vi "QTI Sensor.vi"(8 "error in (no error)":errorcluster, 9 "level":dbl, 11 "IIC in":refnum<class "IIC.lvclass">) -> (0 "error out":errorcluster, 1 "QTI Binary":bool[](array[boolean]), 2 "QTI":dbl[](array[numeric]), 3 "IIC out":refnum<class "IIC.lvclass">)   [LabVIEW 2020]
uses:
  <vilib>/High Genius/HG_WSI_Tookit/Dependencies/Library/IIC/IIC.lvclass
  C:/Program Files (x86)/National Instruments/LabVIEW 2020/vi.lib/High Genius/HG_WSI_Tookit/Dependencies/Library/HG_LIB/HG_LIB.lvclass
  <vilib>/High Genius/HG_WSI_Tookit/Dependencies/Library/HG_LIB/HG_LIB.lvclass
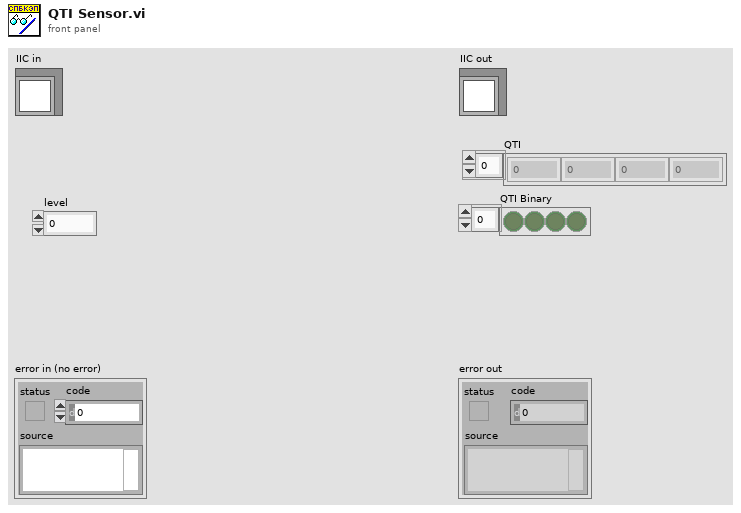
[diagram p1: front panel]
types:
  T1 = cluster{"data":cluster{"ai22":sgl, "ai23":sgl, "ai24":sgl, "ai25":sgl, "pulse12":i32, "pulse13":i32, "pwm14":i32, "pwm15":i32, "pwm16":i32, "do17":bool, "do18":bool, "do19":bool, "do20":bool, "do21":bool, "di11":bool, "di9":bool, "motor0":u8, "motor1":u8, "motor2":u8, "motor3":u8, "dir00":u8, "dir01":u8, "dir02":u8, "dir03":u8, "dir10":u8, "dir11":u8, "dir12":u8, "dir13":u8, "limit0":bool, "limit1":bool, "limit2":bool, "limit3":bool, "limit4":bool, "limit5":bool, "limit6":bool, "limit7":bool, "lsb0H":u8, "lsb1H":u8, "lsb2H":u8, "lsb3H":u8, "lsb0L":u8, "lsb1L":u8, "lsb2L":u8, "lsb3L":u8, "enc0_counters":u32, "enc1_counters":u32, "enc2_counters":u32, "enc3_counters":u32, "counter10":u32, "counter8":u32, "reset_enc0":bool, "reset_enc1":bool, "reset_enc2":bool, "reset_enc3":bool, "pitch":sgl, "roll":sgl, "yaw":sgl, "zero_yaw":bool}}
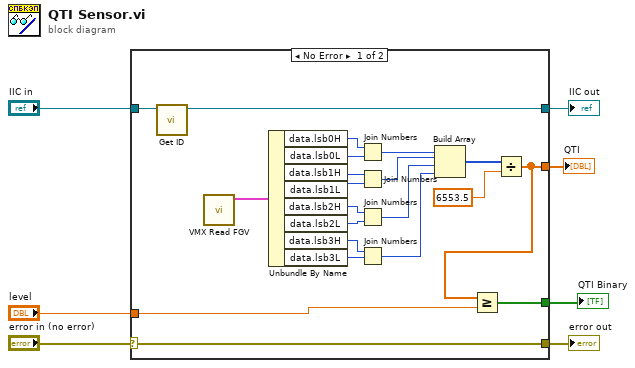
[diagram p0: block diagram]
diagram:
  n1 = case shown="No Error" "error in (no error)" {
    selector: "error in (no error)" -> [w13 w30]
    tunnel: [w13 w30] -> w3
    tunnel: [w28 w29] -> w5
    tunnel: "IIC in" -> [w27 w29]
    tunnel: [w9 _] -> w4
    tunnel: "level" -> [w10 _]
    tunnel: [w8 _] -> w1
    frame No Error {
      n2 = call <vilib>:"Get ID.vi"("HG_LIB in"=w27) -> ("HG_LIB out"=w28:refnum<class "IIC.lvclass">)  [unwired: 9 in, 1 out]
      n3 = call <vilib>:"VMX Read FGV.vi"() -> ("Read Data"=w20:T1)  [unwired: 10 in, 1 out]
      n4 = Unbundle By Name(w20) -> ("data.lsb0H"=w19:u8, "data.lsb0L"=w18:u8, "data.lsb1H"=w17:u8, "data.lsb1L"=w16:u8, "data.lsb2H"=w15:u8, "data.lsb2L"=w14:u8, "data.lsb3H"=w12:u8, "data.lsb3L"=w11:u8)
      n5 = Join Numbers(hi=w19, lo=w18) -> ((hi.lo)=w26:u16)
      n6 = Join Numbers(hi=w17, lo=w16) -> ((hi.lo)=w25:u16)
      n7 = Join Numbers(hi=w15, lo=w14) -> ((hi.lo)=w24:u16)
      n8 = Join Numbers(hi=w12, lo=w11) -> ((hi.lo)=w23:u16)
      n9 = Build Array(w26, w25, w24, w23) -> (w22:u16[])
      n10 = Divide(x=w22, y=6553.5) -> (x/y=w9:dbl[])
      n11 = Greater Or Equal?(x=w9, y=w10) -> (x >= y?=w8:bool[])
    }
    frame Error {
    }
  }
  "error out" <- w3
  "IIC out" <- w5
  "QTI" <- w4
  "QTI Binary" <- w1
